vi "ChildImplementationDefaultValue--Constant.vi"() -> (3 "ChildImplementationDefaultValue":string)   [LabVIEW 2021, in "IconEditorInterface.lvlib" / "IconEditorInterface.lvclass"]
uses:
  <resource>/plugins/NIIconEditor/UI/Interface class/IconEditorInterface.lvclass
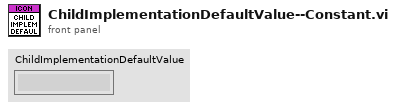
[diagram p1: front panel]
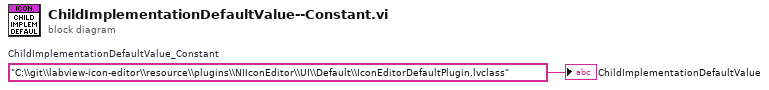
[diagram p0: block diagram]
diagram:
  w1 = "C:\\git\\labview-icon-editor\\resource\\plugins\\NIIconEditor\\UI\\Default\\IconEditorDefaultPlugin.lvclass"  # ChildImplementationDefaultValue_Constant
  "ChildImplementationDefaultValue" <- w1
